vi "PathNotNull.vi"(9 "Path In":path) -> (0 "Not Null Out":bool)   [LabVIEW 2024, in "LVarex.lvlib"]
uses:
  LVarex.lvlib
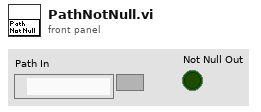
[diagram p1: front panel]
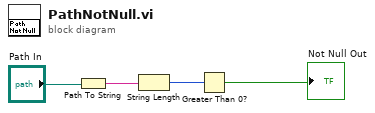
[diagram p0: block diagram]
diagram:
  n1 = Path To String(path="Path In") -> (string=w3:string)
  n2 = String Length(string=w3) -> (length=w2:i32)
  n3 = Greater Than 0?(x=w2) -> (x > 0?=→"Not Null Out":bool)
